vi "Scan Hydra - Cal - Manual.vi"(2 "error in":errorcluster) -> (0 "error out":errorcluster, 1 "next scan":dbl[](array[numeric]) format="%.2f")   [LabVIEW 2019]
uses:
  Global Variables/Global_Variables.vi
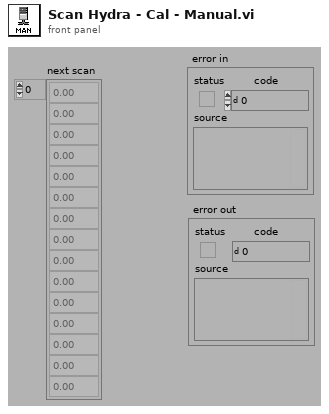
[diagram p1: front panel]
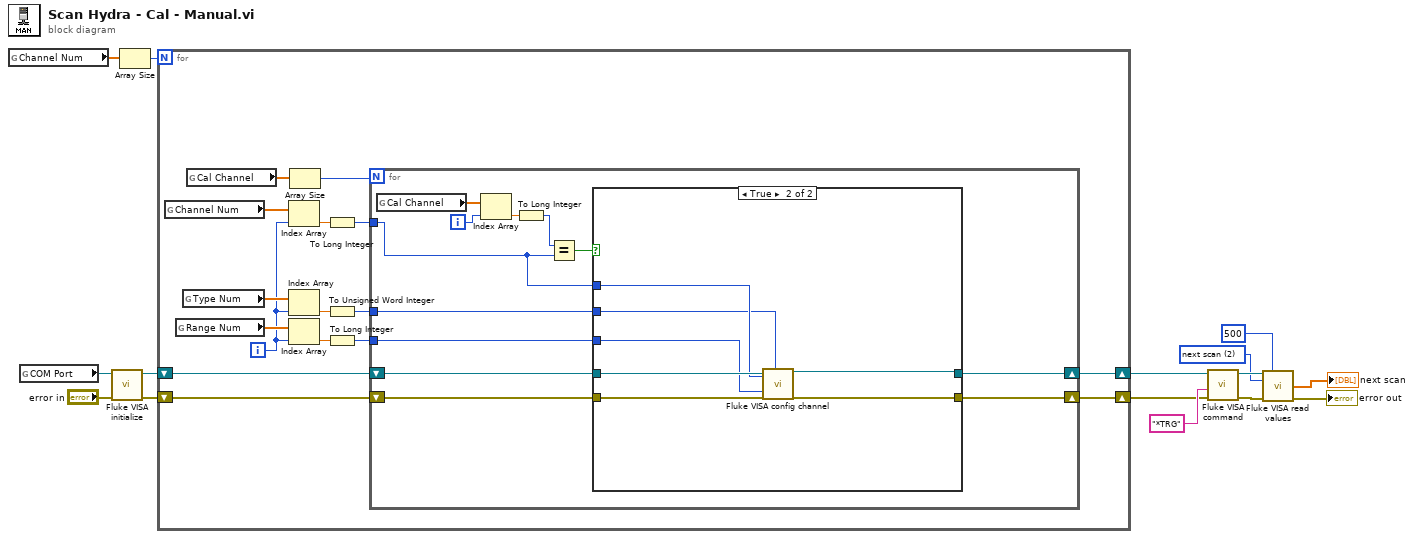
[diagram p0: block diagram]
diagram:
  w10 = 2 items=["min, max, & last", "monitor value", "next scan", "current total"] ("values to read")
  n1 = global read "Global_Variables.vi" "Channel Num"() -> (w6:dbl[])
  n2 = global read "Global_Variables.vi" "COM Port"() -> (w7:refnum<visa-resource-name>)
  n3 = call "Fluke VISA initialize.vi"("error in (no error)"="error in", "Hydra VISA in"=w7) -> ("error out"=w3:errorcluster, "Hydra VISA out"=w4:refnum<visa-resource-name>)  [unwired: 3 in, 1 out]
  n4 = Array Size(array=w6) -> (size(s)=w5:i32)
  n5 = for {
    N: w5 -> [_]
    shift-right: [w19] -> w1
    shift-left: w4 -> [w22]
    shift-right: [w18] -> w2
    shift-left: w3 -> [w21]
    i -> [w28]
    n6 = global read "Global_Variables.vi" "Channel Num"() -> (w31:dbl[])
    n7 = global read "Global_Variables.vi" "Range Num"() -> (w29:dbl[])
    n8 = global read "Global_Variables.vi" "Type Num"() -> (w30:dbl[])
    n9 = global read "Global_Variables.vi" "Cal Channel"() -> (w24:dbl[])
    n10 = Index Array(array=w31, index=w28) -> (element=w27:dbl)
    n11 = Index Array(array=w30, index=w28) -> (element=w26:dbl)
    n12 = Index Array(array=w29, index=w28) -> (element=w25:dbl)
    n13 = Array Size(array=w24) -> (size(s)=w23:i32)
    n14 = To Long Integer(number=w27) -> (32bit integer=w20:i32)
    n15 = To Unsigned Word Integer(number=w26) -> (unsigned 16bit integer=w17:u16)
    n16 = To Long Integer(number=w25) -> (32bit integer=w16:i32)
    n17 = for {
      N: w23 -> [_]
      tunnel: w20 -> [w34]
      shift-right: [w35] -> w19
      shift-left: w22 -> [w37]
      shift-right: [w36] -> w18
      shift-left: w21 -> [w38]
      tunnel: w17 -> [w33]
      tunnel: w16 -> [w32]
      i -> [w42]
      n18 = global read "Global_Variables.vi" "Cal Channel"() -> (w43:dbl[])
      n19 = Index Array(array=w43, index=w42) -> (element=w41:dbl)
      n20 = To Long Integer(number=w41) -> (32bit integer=w40:i32)
      n21 = Equal?(x=w40, y=w34) -> (x = y?=w39:bool)
      n22 = case shown="True" w39 {
        tunnel: w38 -> [w45 w52]
        tunnel: w37 -> [w44 w50]
        tunnel: [w45 w51] -> w36
        tunnel: [w44 w49] -> w35
        tunnel: w34 -> [_ w48]
        tunnel: w33 -> [_ w47]
        tunnel: w32 -> [_ w46]
        frame False {
        }
        frame True {
          n23 = call "Fluke VISA config channel.vi"("Hydra VISA in"=w50, "channel"=w48, "range (auto:0)"=w46, "error in (no error)"=w52, "function (off:0)"=w47) -> ("Hydra VISA out"=w49:refnum<visa-resource-name>, "error out"=w51:errorcluster)  [unwired: 13 in]
        }
      }
    }
  }
  n24 = call "Fluke VISA command.vi"("error in (no error)"=w2, "Single Command"="*TRG", "Hydra VISA in"=w1) -> ("error out"=w13:errorcluster, "Hydra VISA out"=w14:refnum<visa-resource-name>)  [unwired: 3 in, 2 out]
  n25 = call "Fluke VISA read values.vi"("Hydra VISA in"=w14, "Byte Count"=u32 500, "values to read"=w10, "error in (no error)"=w13) -> ("next scan"=→"next scan":dbl[], "error out"=→"error out":errorcluster)  [unwired: 4 in, 6 out]
